vi "Handle Data.vi"(8 "error in (no error)":errorcluster, 10 "Data":dbl, 11 "ChartProc in":refnum<class "ChartProc.lvclass">) -> (0 "error out":errorcluster, 3 "ChartProc out":refnum<class "ChartProc.lvclass">)   [LabVIEW 2020, in "LAF2024Q2.lvlib" / "ChartProc.lvclass"]
uses:
  ChartProc.lvclass
  ChartProc.lvclass/ChartProc.ctl
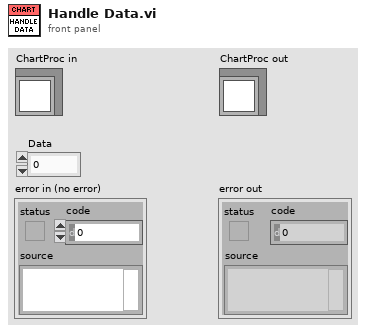
[diagram p1: front panel]
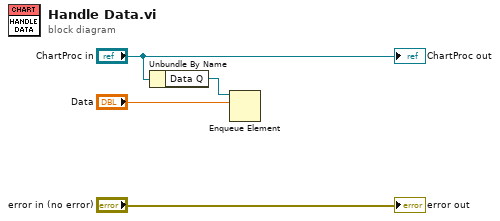
[diagram p0: block diagram]
diagram:
  n1 = Unbundle By Name("ChartProc in") -> ("Data Q"=w2:refnum<queue>)
  n2 = Enqueue Element(queue=w2, element="Data") -> ()  [unwired: 2 in, 3 out]
  "error out" <- "error in (no error)"
  "ChartProc out" <- "ChartProc in"
